vi "MainConfig.vi"(10 "Plugin info":T3, 11 "Input Data":T1={"BasePath"=path "C:/CustomDashboard/MainConfig", "CommunicationData"={"TargetFilePath"="/media/sda1", "ConnectionData"={"host"="roborio-223-frc.local", "user"="lvuser", "password"="", "port"=22}}}) -> ()   [LabVIEW 2016]
uses:
  General/CorePluginInfo.ctl
  ConfigXML/typedefs/ConfigXMLInputData.ctl
  General/RemoteFiles/connectionData.ctl
  ConfigXML/typedefs/OmniHButterfly.ctl
  ConfigXML/typedefs/DriveSide.ctl
  ConfigXML/typedefs/MotorControl.ctl
  ConfigXML/typedefs/EncoderControl.ctl
  ConfigXML/typedefs/PIDControl.ctl
  ConfigXML/typedefs/Solenoid.ctl
  ConfigXML/src/ConfigXMLControl.ctl
panel:
  in  "ViewConfigText":bool
  out "Config Currently on Target":string
  out "windowName":string
  in  "ViewCfgOnBot":bool
  in  "ULConfigtoRIO":bool
  in  "LoadConfig":bool
  in  "SaveConfig":bool
  in  "Tab Control":T4(tab)
  in  "Drive":T5
  in  "Shooter":T11
  in  "Gear":T12
  in  "Hangar":cluster{"motor":T7}
  in  "Intake":cluster{"motor":T7}
  in  "debugPin":i32
  in  "VisionServer":cluster{"address":string, "port":i32}
  in  "pdpID":dbl
  in  "DEBUG":bool
  in  "auto":T13
  # "NOTE: All encoder / PID info assumes traction wheels, and is \nmultiplied / divided by omniReductionScalar for omni wheels"
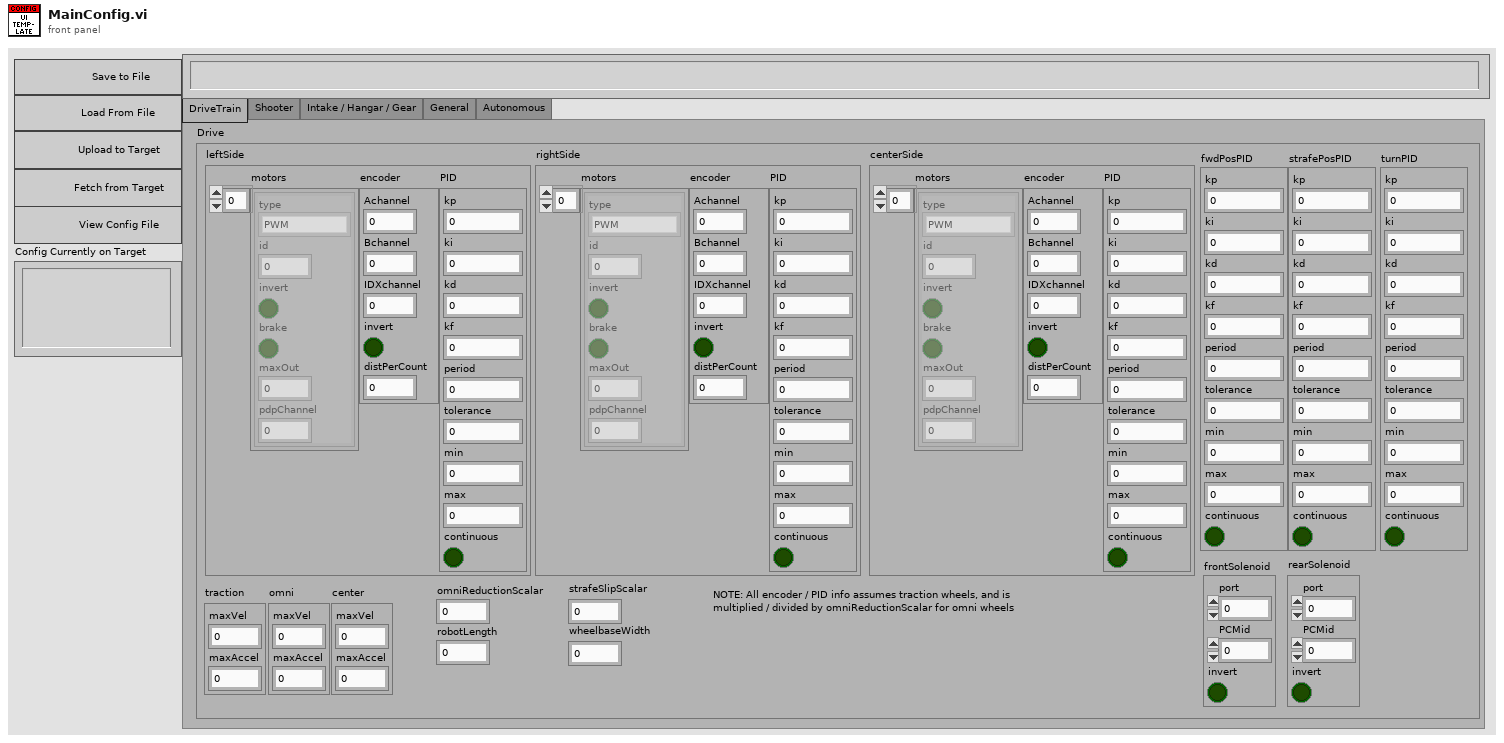
[diagram p1: front panel]
types:
  T1 = typedef "ConfigXMLInputData.ctl" = cluster{"BasePath":path, "CommunicationData":cluster{"TargetFilePath":string, "ConnectionData":T2}}
  T2 = typedef "connectionData.ctl" = cluster{"host":string, "user":string, "password":string, "port":u16}
  T3 = typedef "CorePluginInfo.ctl" = cluster{"Notifiers":cluster{"Robot IP Notifier":refnum<notifier>, "Window Mode Notifier":refnum<notifier>, "Stop Notifier":refnum<notifier>}}
  T4 = enum32{"DriveTrain", "Shooter", "Intake / Hangar / Gear", "General", "Autonomous"}
  T5 = typedef "OmniHButterfly.ctl" = cluster{"leftSide":T6, "rightSide":T6, "centerSide":T6, "fwdPosPID":T9, "strafePosPID":T9, "turnPID":T9, "frontSolenoid":T10, "rearSolenoid":T10, "traction":cluster{"maxVel":dbl, "maxAccel":dbl}, "omni":cluster{"maxVel":dbl, "maxAccel":dbl}, "center":cluster{"maxVel":dbl, "maxAccel":dbl}, "strafeSlipScalar":dbl, "wheelbaseWidth":dbl, "omniReductionScalar":dbl, "robotLength":dbl}
  T6 = typedef "DriveSide.ctl" = cluster{"motors":T7[], "encoder":T8, "PID":T9}
  T7 = typedef "MotorControl.ctl" = cluster{"type":enum16{"PWM", "CANTalon"}, "id":i32, "invert":bool, "brake":bool, "maxOut":dbl, "pdpChannel":i32}
  T8 = typedef "EncoderControl.ctl" = cluster{"Achannel":i32, "Bchannel":i32, "IDXchannel":i32, "invert":bool, "distPerCount":dbl}
  T9 = typedef "PIDControl.ctl" = cluster{"kp":dbl, "ki":dbl, "kd":dbl, "kf":dbl, "period":dbl, "tolerance":dbl, "min":dbl, "max":dbl, "continuous":bool}
  T10 = typedef "Solenoid.ctl" = cluster{"port":i32, "PCMid":i32, "invert":bool}
  T11 = cluster{"wheels":cluster{"motor":T7, "encoder":T8, "PID":T9, "targetSpeed":dbl}, "auger":cluster{"motor":T7, "encoder":T8, "PID":T9}}
  T12 = cluster{"dropTime":dbl, "puncher":T10, "jaws":T10}
  T13 = cluster{"mode":enum16{"crossLine", "boiler", "gear1", "gear2", "gear3", "doNothing"}, "gear1":cluster{"fwdDist":dbl, "approachDist":dbl, "lineCrossDist":dbl}, "general":cluster{"crossLineAfter":bool, "towerDist":dbl, "towerAngle":dbl, "towerWidth":dbl}, "gear3":cluster{"fwdDist":dbl, "approachDist":dbl, "lineCrossDist":dbl}, "gear2":cluster{"approachDist":dbl}, "boiler":cluster{"strafeDist":dbl, "turnAngle":dbl}}
  T14 = typedef "ConfigXMLControl.ctl" = cluster{"ViewCfgOnTarget":refnum<vi>, "ULConfigtoTarget":refnum<vi>, "TabControl":refnum<vi>, "ConfigOnTarget":refnum<vi>, "LoadConfig":refnum<vi>, "SaveConfig":refnum<vi>, "BaseDirectory":path, "TargetFilePath":string, "ViewConfigText":refnum<vi>, "Plugin Info":T3}
  T15 = cluster{"TargetFilePath":string, "ConnectionData":T2}
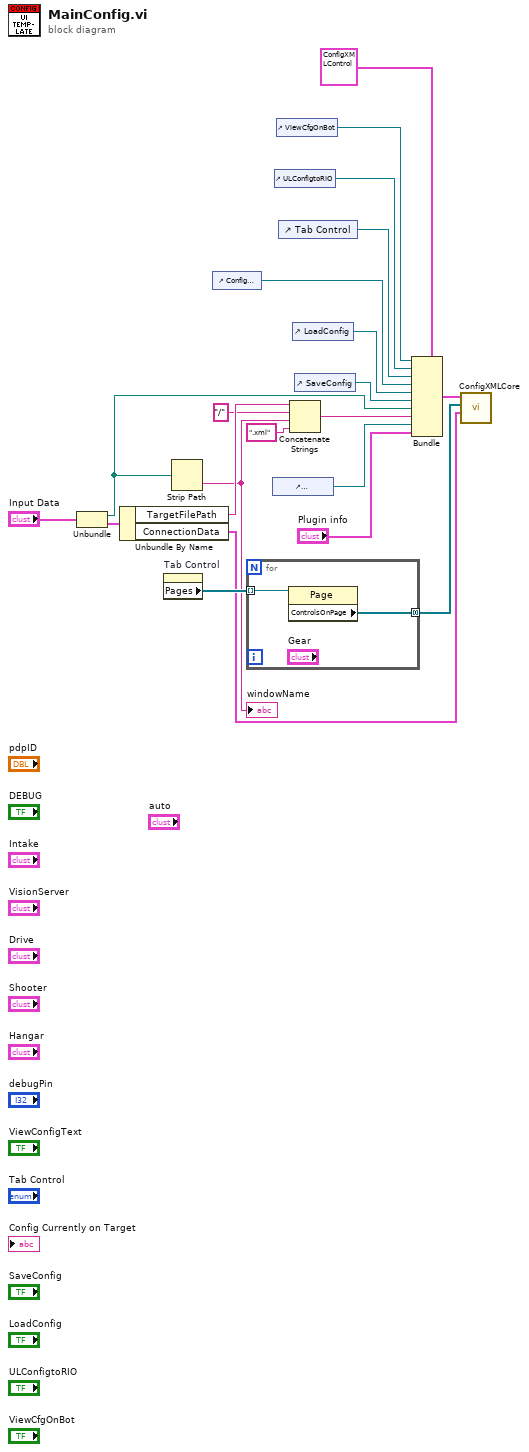
[diagram p0: block diagram]
diagram:
  n1 = Unbundle("Input Data") -> ("BasePath"=w2:path, "CommunicationData"=w1:T15)
  n2 = Unbundle By Name(w1) -> ("TargetFilePath"=w10:string, "ConnectionData"=w11:T2)
  n3 = property on="Tab Control" class="TabCtl (strict)"() -> ("Pages"=w21:refnum<vi>[])  [unwired: 2 in, 2 out]
  n4 = Strip Path(path=w2) -> (name=w8:string)  [unwired: 1 out]
  "windowName" <- w8
  n5 = control-ref of="Config Currently on Target"() -> (w13:refnum<vi>)
  n6 = for {
    tunnel: w21 -> [w23] mode=indexing
    tunnel: [w22] -> w14 mode=concatenating
    n7 = property class="Page"(reference=w23) -> ("ControlsOnPage"=w22:refnum<vi>[])  [unwired: 1 in, 2 out]
  }
  n8 = control-ref of="ViewConfigText"() -> (w5:refnum<vi>)
  n9 = control-ref of="ULConfigtoRIO"() -> (w19:refnum<vi>)
  n10 = control-ref of="ViewCfgOnBot"() -> (w20:refnum<vi>)
  n11 = control-ref of="Tab Control"() -> (w12:refnum<vi>)
  n12 = Concatenate Strings(w10, "/" ("string"), w8, ".xml" ("string")) -> (w6:string)
  n13 = control-ref of="LoadConfig"() -> (w18:refnum<vi>)
  n14 = control-ref of="SaveConfig"() -> (w17:refnum<vi>)
  n15 = Bundle(cluster=T14 {"ViewCfgOnTarget"=refnum, "ULConfigtoTarget"=refnum, "TabControl"=refnum, "ConfigOnTarget"=refnum, "LoadConfig"=refnum, "SaveConfig"=refnum, "BaseDirectory"=path "", "TargetFilePath"="", "ViewConfigText"=refnum, "Plugin Info"={"Notifiers"={"Robot IP Notifier"=refnum, "Window Mode Notifier"=refnum, "Stop Notifier"=refnum}}} ("output cluster"), "ViewCfgOnTarget"=w20, "ULConfigtoTarget"=w19, "TabControl"=w12, "ConfigOnTarget"=w13, "LoadConfig"=w18, "SaveConfig"=w17, "BaseDirectory"=w2, "TargetFilePath"=w6, "ViewConfigText"=w5, "Plugin Info"="Plugin info") -> (w15:T14)
  n16 = call "ConfigXMLCore.vi"("ConnectionData"=w11, "controlsToSave"=w14, "ConfigXMLControl"=w15) -> ()  [unwired: 9 in]
